vi "GROM_GUI_calc_coords.vi"(9 "corr amps":T1, 10 "amps":T2={"number"=0, "type"=0, "rotated"=0, "fliped"=0, "FPAcoord"={"xstart"=1, "ystart"=1}, "Physical_size"={"columns"=0, "rows"=0}, "predata"={"columns"=0, "rows"=0}, "postdata"={"columns"=0, "rows"=0}, "Req ROIs"=[], "Corr ROI"=[], "Detnumber"=0, "ampID"="", "discard"=0} {"fliped" items=["none", "horizontal", "vertical"]; "type" items=["LL", "LR", "UL", "UR"]}) -> (1 "virt coords":string, 2 "phys coords":string)   [LabVIEW 2016]
uses:
  private/vis/GEOM_Amplifier.ctl
  private/vis/GEOM_AmpType.ctl
  private/vis/GEOM_ROI.ctl
  private/vis/GEOM_Coords.ctl
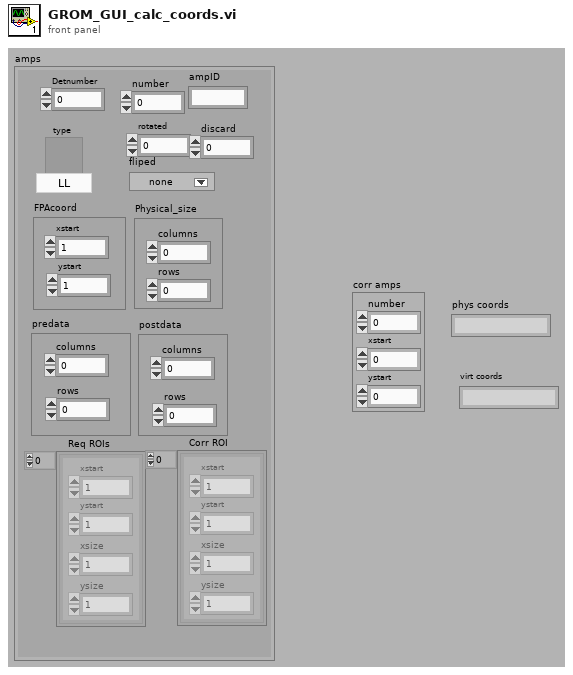
[diagram p1: front panel]
types:
  T1 = cluster{"number":i32, "xstart":i32, "ystart":i32}
  T2 = typedef "GEOM_Amplifier.ctl" = cluster{"number":i32, "type":T3, "rotated":i16, "fliped":u16, "FPAcoord":cluster{"xstart":i32, "ystart":i32}, "Physical_size":cluster{"columns":i32, "rows":i32}, "predata":cluster{"columns":i32, "rows":i32}, "postdata":cluster{"columns":i32, "rows":i32}, "Req ROIs":T4, "Corr ROI":T4, "Detnumber":i32, "ampID":string, "discard":i32}
  T3 = typedef "GEOM_AmpType.ctl" = u16
  T4 = typedef "GEOM_ROI.ctl" = T5[]
  T5 = typedef "GEOM_Coords.ctl" = cluster{"xstart":u32, "ystart":u32, "xsize":u32, "ysize":u32}
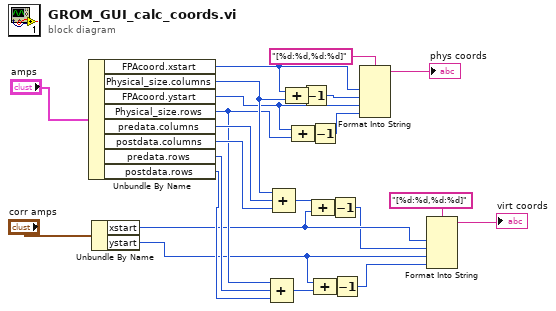
[diagram p0: block diagram]
diagram:
  n1 = Unbundle By Name("amps") -> ("FPAcoord.xstart"=w16:i32, "Physical_size.columns"=w15:i32, "FPAcoord.ystart"=w12:i32, "Physical_size.rows"=w11:i32, "predata.columns"=w21:i32, "postdata.columns"=w20:i32, "predata.rows"=w19:i32, "postdata.rows"=w18:i32)
  n2 = Unbundle By Name("corr amps") -> ("xstart"=w6:i32, "ystart"=w2:i32)
  n3 = Compound Arithmetic op=ADD(w11, w19, w18) -> (w3:i32)
  n4 = Compound Arithmetic op=ADD(w15, w21, w20) -> (w7:i32)
  n5 = Compound Arithmetic op=ADD(w16, w15) -> (w14:i32)
  n6 = Compound Arithmetic op=ADD(w12, w11) -> (w10:i32)
  n7 = Decrement(x=w14) -> (x-1=w13:i32)
  n8 = Decrement(x=w10) -> (x-1=w9:i32)
  n9 = Compound Arithmetic op=ADD(w7, w6) -> (w8:i32)
  n10 = Compound Arithmetic op=ADD(w2, w3) -> (w4:i32)
  n11 = Decrement(x=w8) -> (x-1=w5:i32)
  n12 = Decrement(x=w4) -> (x-1=w1:i32)
  n13 = Format Into String(format string="[%d:%d,%d:%d]", w16, w13, w12, w9) -> (resulting string=→"phys coords":string)  [unwired: 2 in, 1 out]
  n14 = Format Into String(format string="[%d:%d,%d:%d]", w6, w5, w2, w1) -> (resulting string=→"virt coords":string)  [unwired: 2 in, 1 out]
